vi "Field Not Supported.vi"(8 "error in":errorcluster, 10 "Field name":string, 11 "Object Type in":refnum<class "Object Type Base.lvclass">) -> (0 "error out":errorcluster)   [LabVIEW 2024, in "EDS.lvlib" / "Object Type Base.lvclass"]
uses:
  Object Type Base.lvclass
  Object Type Base.lvclass/Object Type Base.ctl
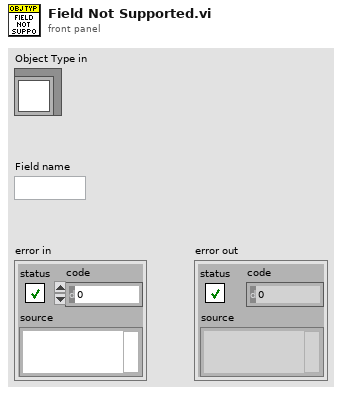
[diagram p1: front panel]
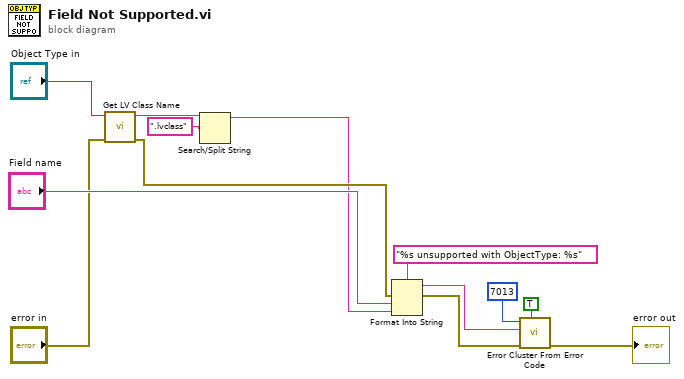
[diagram p0: block diagram]
diagram:
  n1 = call <vilib>:"Get LV Class Name.vi"("error in (no error)"="error in", "object"="Object Type in") -> ("error out"=w3:errorcluster, "class name"=w6:string)  [unwired: 8 in]
  n2 = Search/Split String(string=w6, search string/char (-)=".lvclass") -> (substring before match=w1:string)  [unwired: 1 in, 2 out]
  n3 = Format Into String(format string="%s unsupported with ObjectType: %s", error in=w3, "Field name", w1) -> (resulting string=w9:string, error out=w2:errorcluster)  [unwired: 1 in]
  n4 = call <vilib>:"Error Cluster From Error Code.vi"("show call chain? (False)"=TRUE, "error in (no error)"=w2, "error message (\"\")"=w9, "error code (0)"=7013) -> ("error out"=→"error out":errorcluster)  [unwired: 5 in]
